vi "Shooter Immediate.vi"(6 "Operation":T1=enum."Immediate", 8 "Flywheel":dbl, 9 "AA?":bool, 10 "Hood":dbl, 11 "Manual Addition":dbl) -> ()   [LabVIEW 2019]
uses:
  <vilib>/Rock Robotics/WPI/Framework/Command Status Info.ctl
  <vilib>/Rock Robotics/WPI/Framework/Completion Status.ctl
  <vilib>/Rock Robotics/WPI/Framework/Completion Notifier.ctl
  Implementation/Shooter Operations.ctl
  Implementation/Shooter Setpoints.ctl
panel:
  in  "Description":string
  out "Command Info Out":T2
  in  "Command Info In":T2
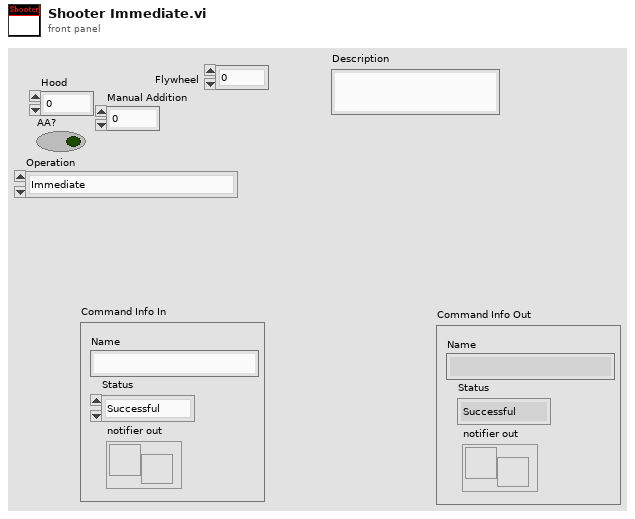
[diagram p1: front panel]
types:
  T1 = typedef "Shooter Operations.ctl" = enum16{"Reserve", "Read Current", "Immediate", "Shoot"}
  T2 = typedef "Command Status Info.ctl" = cluster{"Name":string, "Status":T3, "notifier out":T4}
  T3 = typedef "Completion Status.ctl" = enum16{"Successful", "Aborted", "Incomplete"}
  T4 = typedef "Completion Notifier.ctl" = refnum<notifier>
  T5 = typedef "Shooter Setpoints.ctl" = cluster{"Operation":T1, "Flywheel":dbl, "Hood":dbl, "AA?":bool, "Manual Addition":dbl}
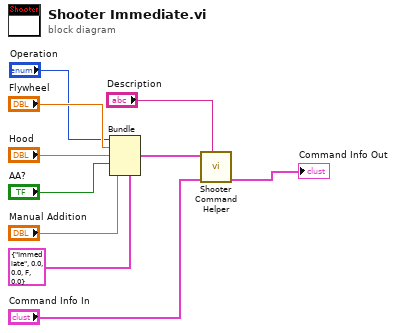
[diagram p0: block diagram]
diagram:
  n1 = Bundle(cluster=T5 {"Operation"=enum."Immediate", "Flywheel"=0.0, "Hood"=0.0, "AA?"=FALSE, "Manual Addition"=0.0} ("SubSystem Data"), "Operation"="Operation", "Flywheel"="Flywheel", "Hood"="Hood", "AA?"="AA?", "Manual Addition"="Manual Addition") -> (w5:T5)
  n2 = call "Shooter Command Helper.vi"("Description"="Description", "Command Info In"="Command Info In", "SubSystem Data"=w5) -> ("Command Info Out"=→"Command Info Out":T2)  [unwired: 6 in, 2 out]
